vi "niP2P Link Peer to Peer Stream.vi"(0 "stream session":refnum<k20>, 11 "error in (no error)":errorcluster) -> (4 "stream session out":refnum<k20>, 15 "error out":errorcluster)   [LabVIEW 2010]
doc: "Links the writer and reader in the stream you specify."
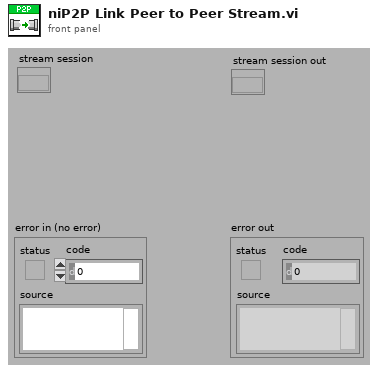
[diagram p1: front panel]
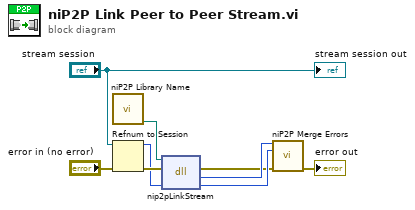
[diagram p0: block diagram]
diagram:
  n1 = call <vilib>:"niP2P Library Name.vi"() -> ("nip2p libname"=w2:path)  [unwired: 10 in]
  n2 = Refnum to Session(4:"error in (no error)", 7:"stream session") -> (0:w9:errorcluster, 3:w7:u64)
  n3 = dll-call lib="?" fn="nip2pLinkStream"(path in=w2, error in=w9, "streamHandle"=w7) -> (error out=w1:errorcluster, "return type"=w4:i32, "streamHandle"=w3:u32)  [unwired: 1 in, 1 out]
  n4 = call <vilib>:"niP2P Merge Errors.vi"("error code"=w4, "stream handle (0)"=w3, "error in"=w1) -> ("error out"=→"error out":errorcluster)  [unwired: 12 in]
  "stream session out" <- "stream session"
